vi "ANAL_TempSummer.vi"(8 "Target Set Points":i32[](array[numeric]), 9 "Software Gate":cluster{"Numeric":i32, "Numeric":i32}, 10 "AorB":bool, 11 "Run Data Cluster":T2 {"Temperature B" scale=0.0..100.0; "Temperature A" scale=0.0..100.0}) -> (2 "Temp Array":T1(array[cluster]))   [LabVIEW 2021]
uses:
  DAT_Cluster.ctl
  503151d4-9f11-43da-a154-24c7c19724c7.vi
  503151d4-9f11-43da-a154-24c7c19724c7.vi/d4db2432-cc9c-482c-8957-dac855435ef6.vi
  503151d4-9f11-43da-a154-24c7c19724c7.vi/86fbf154-bd7b-49a2-8ab2-a837b2a95f24.vi
  503151d4-9f11-43da-a154-24c7c19724c7.vi/3b95b01e-1ec2-4565-bcd9-7606a5281010.vi
  503151d4-9f11-43da-a154-24c7c19724c7.vi/96a08935-737a-44b2-979c-a81d56408f7e.vi
  503151d4-9f11-43da-a154-24c7c19724c7.vi/d4db2432-cc9c-482c-8957-dac855435ef6.vi/6eaecd13-6e48-4772-a921-b51ebdf84d88.vi
  503151d4-9f11-43da-a154-24c7c19724c7.vi/d4db2432-cc9c-482c-8957-dac855435ef6.vi/d2d5f2b7-06f4-47f6-971c-049c3fdbb653.vi
  503151d4-9f11-43da-a154-24c7c19724c7.vi/3b95b01e-1ec2-4565-bcd9-7606a5281010.vi/6eaecd13-6e48-4772-a921-b51ebdf84d88.vi
  503151d4-9f11-43da-a154-24c7c19724c7.vi/3b95b01e-1ec2-4565-bcd9-7606a5281010.vi/d2d5f2b7-06f4-47f6-971c-049c3fdbb653.vi
  503151d4-9f11-43da-a154-24c7c19724c7.vi/96a08935-737a-44b2-979c-a81d56408f7e.vi/6eaecd13-6e48-4772-a921-b51ebdf84d88.vi
  503151d4-9f11-43da-a154-24c7c19724c7.vi/96a08935-737a-44b2-979c-a81d56408f7e.vi/d2d5f2b7-06f4-47f6-971c-049c3fdbb653.vi
  <vilib>/Comparison/Less/Less Functor/Less Functor.lvclass
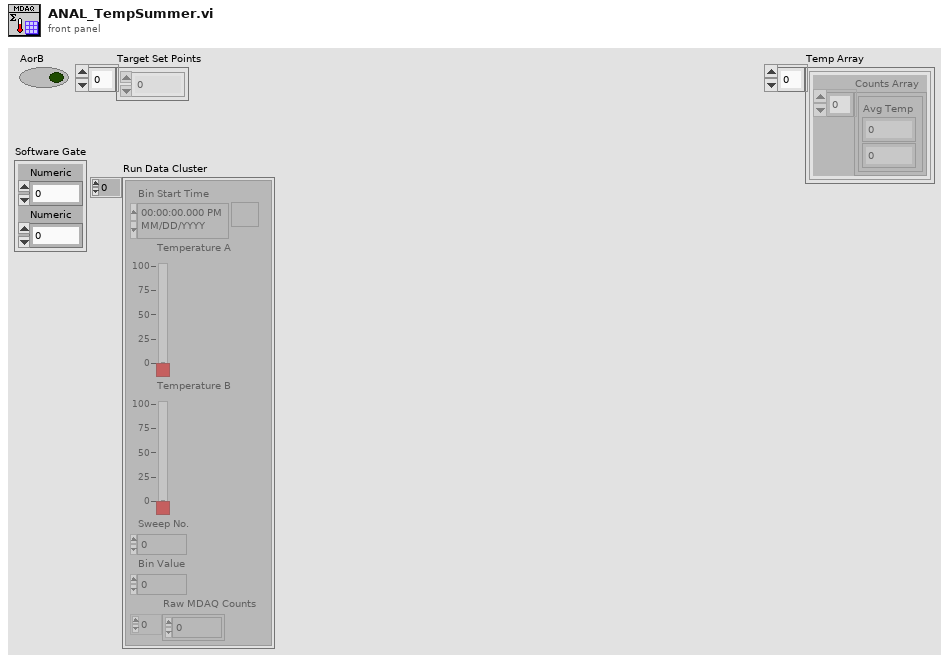
[diagram p1: front panel]
types:
  T1 = cluster{"Counts Array":cluster{"Avg Temp":dbl, i32}[]}[]
  T2 = typedef "DAT_Cluster.ctl" = cluster{"Bin Start Time":timestamp, "Temperature A":dbl, "Temperature B":dbl, "Sweep No.":i32, "Bin Value":i32, "Raw MDAQ Counts":i32[]}[]
  T3 = cluster{"Counts Array":cluster{"Avg Temp":dbl, i32}[]}
  T4 = cluster{"Temperature B":dbl, "Numeric":i32, "nearest index":i32}[]
  T5 = cluster{"Temperature B":dbl, "Numeric":i32, "nearest index":i32}
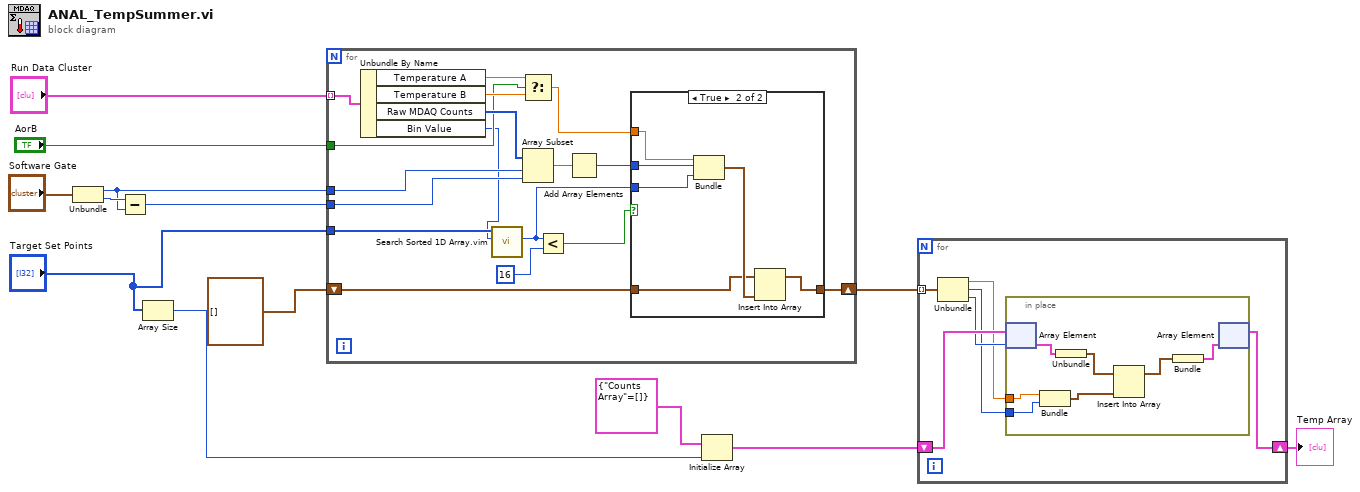
[diagram p0: block diagram]
diagram:
  n1 = Unbundle("Software Gate") -> ("Numeric"=w10:i32, "Numeric"=w11:i32)
  n2 = Subtract(x=w11, y=w10) -> (x-y=w9:i32)
  n3 = Array Size(array="Target Set Points") -> (size(s)=w4:i32)
  n4 = for {
    tunnel: "Run Data Cluster" -> [w30] mode=indexing
    tunnel: w10 -> [w28]
    tunnel: w9 -> [w27]
    tunnel: "AorB" -> [w23]
    tunnel: "Target Set Points" -> [w21]
    shift-right: [w15] -> w5
    shift-left: T4 [] -> [w14]
    n5 = Unbundle By Name(w30) -> ("Temperature A"=w25:dbl, "Temperature B"=w24:dbl, "Raw MDAQ Counts"=w29:i32[], "Bin Value"=w20:i32)
    n6 = call "Search Sorted 1D Array.vim"("element"=w20, "sorted 1D array"=w21) -> ("nearest index"=w17:i32)  [unwired: 8 in, 1 out]
    n7 = Select(t=w25, s=w23, f=w24) -> (s? t:f=w19:dbl)
    n8 = Array Subset(array=w29, index=w28, length=w27) -> (w26:i32[])
    n9 = Less?(x=w17, y=16) -> (x < y?=w16:bool)
    n10 = Add Array Elements(numeric array=w26) -> (sum=w18:i32)
    n11 = case shown="True" w16 {
      tunnel: w19 -> [_ w37]
      tunnel: w18 -> [_ w36]
      tunnel: w17 -> [_ w35]
      tunnel: [w31 w33] -> w15
      tunnel: w14 -> [w31 w32]
      frame False {
      }
      frame True {
        n12 = Bundle("Temperature B"=w37, "Numeric"=w36, "nearest index"=w35) -> (w34:T5)  [unwired: 1 in]
        n13 = Insert Into Array(array=w32, new element=w34) -> (w33:T4)  [unwired: 1 in]
      }
    }
  }
  n14 = Initialize Array(T3 {"Counts Array"=[]}, w4) -> (w2:T1)
  n15 = for {
    tunnel: w5 -> [w43] mode=indexing
    shift-right: [w38] -> w1
    shift-left: w2 -> [w42]
    n16 = Unbundle(w43) -> ("Temperature B"=w39:dbl, "Numeric"=w40:i32, "nearest index"=w41:i32)
    n17 = in-place {
      in-place-border: w40 -> [w45]
      in-place-border: w39 -> [w46]
      n18 = in-place-array #1(w42, w41) -> (w50:T3)
      n19 = Bundle("Temperature B"=w46, "Numeric"=w45) -> (w44:cluster{"Temperature B":dbl, "Numeric":i32})  [unwired: 1 in]
      n20 = Unbundle(w50) -> ("Counts Array"=w49:cluster{"Avg Temp":dbl, i32}[])
      n21 = Insert Into Array(array=w49, new element=w44) -> (w48:cluster{"Avg Temp":dbl, i32}[])  [unwired: 1 in]
      n22 = Bundle("Counts Array"=w48) -> (w47:T3)  [unwired: 1 in]
      n23 = in-place-array #1(w47) -> (w38:T1)  [unwired: 1 out]
    }
  }
  "Temp Array" <- w1
